vi "TGC.vi"(0 "System no.":i32=1 min=1 max=4 step=1, 2 "Trajectory ID":i32[](array[numeric]), 5 "error in":errorcluster) -> (19 "error out":errorcluster)   [LabVIEW 2026]
doc: "Clear all values of trajectories. For further details, see Trajectories for Motion Paths in the controller user manual.\n\nC-867, C-884:"
panel:
  # "Clear all values of trajectories."
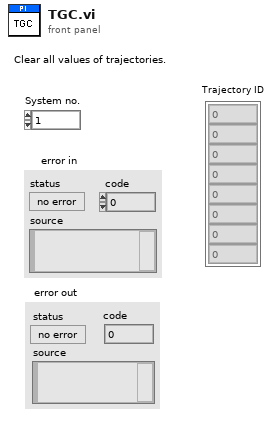
[diagram p1: front panel]
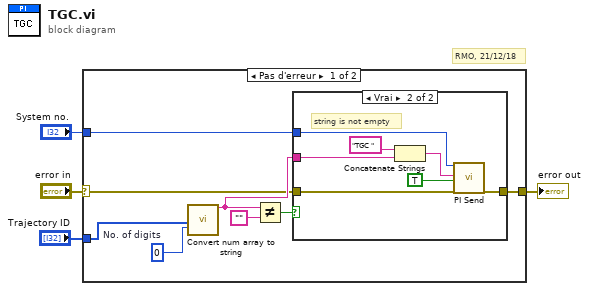
[diagram p0: block diagram]
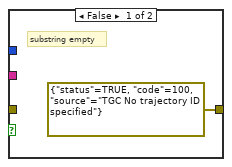
[diagram p2: hidden frame]
diagram:
  # "RMO, 21/12/18"
  n1 = case shown="Pas d'erreur" "error in" {
    selector: "error in" -> [w5 w21]
    tunnel: [w12 w21] -> w4
    tunnel: "System no." -> [w10 _]
    tunnel: "Trajectory ID" -> [w8 _]
    frame No Error {
      w6 = i16 0  # No. of digits
      n2 = call "Convert num array to string.vi"("Num. values"=w8, "No. of digits"=w6) -> ("Output string"=w7:string)  [unwired: 17 out]
      n3 = Not Equal?(x=w7, y="") -> (x != y?=w9:bool)
      n4 = case shown="Vrai" w9 {
        tunnel: w7 -> [_ w19]
        tunnel: [errorcluster {"status"=TRUE, "code"=100, "source"="TGC No trajectory ID specified"} ("error out") w15] -> w12
        tunnel: w5 -> [_ w16]
        tunnel: w10 -> [_ w14]
        frame False {
          # "substring empty"
        }
        frame True {
          # "string is not empty"
          n5 = Concatenate Strings("TGC ", w19) -> (w17:string)
          n6 = call "PI Send.vi"("System no."=w14, "String to send"=w17, "Attach termination char.?"=TRUE ("Attach Linefeed?"), "error in"=w16) -> ("error out"=w15:errorcluster)  [unwired: 2 in, 13 out]
        }
      }
    }
    frame Error {
    }
  }
  "error out" <- w4
